vi "init.vi"(8 "error in (no error)":errorcluster, 11 "Thermocouples in":refnum<class "Thermocouples.lvclass">) -> (0 "error out":errorcluster, 3 "Thermocouples out":refnum<class "Thermocouples.lvclass">)   [LabVIEW 2025, in "Thermocouples.lvclass"]
uses:
  Thermocouples.lvclass
  Thermocouples.lvclass/Thermocouples.ctl
  <vilib>/DAQmx/create/channels.llb/DAQmx Create Channel (AI-Temperature-Thermocouple).vi
panel:
  in  "units":i32(ring)=10144 items=["Deg C"=10143, "Deg F"=10144, "Kelvins"=10325, "Deg R"=10145, "From Custom Scale"=10065]
  in  "cjc value":dbl=72.0 format="%0.2f"
  in  "T/C Type [K]":i32(ring)=10073 items=["J"=10072, "K"=10073, "N"=10077, "R"=10082, "S"=10085, "T"=10086, "B"=10047, "E"=10055]
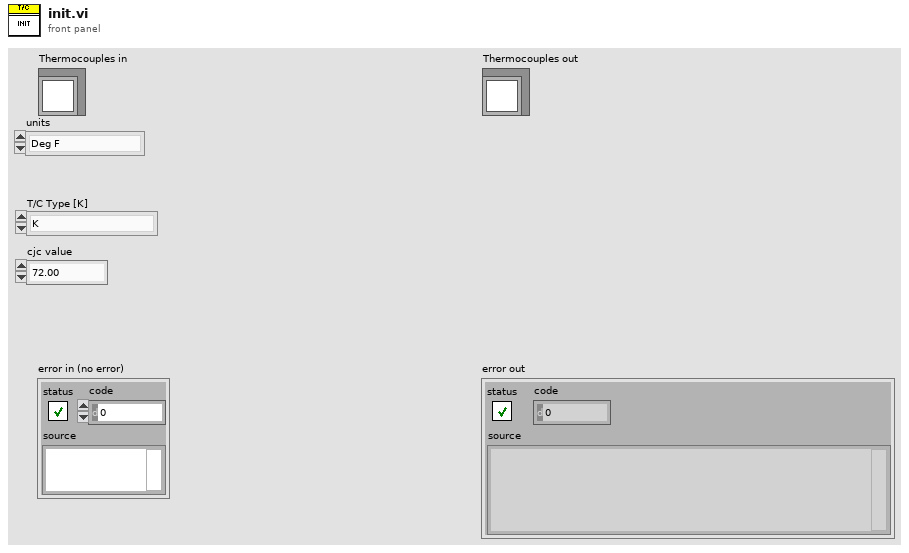
[diagram p1: front panel]
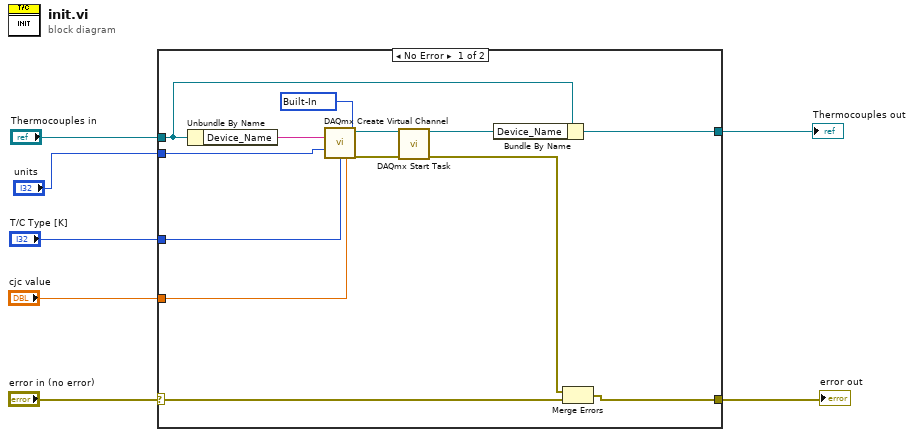
[diagram p0: block diagram]
diagram:
  n1 = case shown="No Error" "error in (no error)" {
    selector: "error in (no error)" -> [w11 w22]
    tunnel: [w9 w22] -> w6
    tunnel: "Thermocouples in" -> [w13 w21]
    tunnel: "T/C Type [K]" -> [w19 _]
    tunnel: "cjc value" -> [w18 _]
    tunnel: [w12 w21] -> w2
    tunnel: "units" -> [w8 _]
    frame No Error {
      w17 = 10200 items=["Built-In"=10200, "Constant Value"=10116, "Channel"=10113] ("cjc source")
      n2 = Unbundle By Name(w13) -> ("Device_Name"=w20:string)
      n3 = call-poly <vilib>:"DAQmx Create Virtual Channel.vi"("physical channels"=w20, "cjc source"=w17, "units"=w8, "thermocouple type"=w19, "cjc value"=w18) -> ("task out"=w16:refnum<k21>, "error out"=w15:errorcluster)  [unwired: 9 in]
      n4 = call <vilib>:"DAQmx Start Task.vi"("task/channels in"=w16, "error in"=w15) -> ("task out"=w14:refnum<k21>, "error out"=w10:errorcluster)  [unwired: 12 in]
      n5 = Bundle By Name(cluster=w13, "Device_Name"=w14) -> (w12:refnum<class "Thermocouples.lvclass">)
      n6 = Merge Errors(w10, w11) -> (w9:errorcluster)
    }
    frame Error {
    }
  }
  "error out" <- w6
  "Thermocouples out" <- w2
